vi "SLSC_Engine Get Module Name.vi"(6 "Connect timeout (s)":dbl, 8 "error in (no error)":errorcluster, 10 "compiled.settings":T2={"Name"="", "SLSC Name or IP Address"="", "Slot #"=0, "Configuration Data"={"Properties"={"Boolean Properties"=[], "Double Properties"=[], "I32 Properties"=[], "I64 Properties"=[], "String Properties"=[], "U32 Properties"=[], "U64 Properties"=[]}, "Commands"=[], "Reset Commands"=[], "Apply Values on Deployment"=TRUE, "Apply Reset on Undeployment"=TRUE, "Change Commands"=[]}, "SLSC Get/Read Properties"=[], "SLSC Set/Write Properties"=[], "SLSC Dynamic Commands"=[], "Support Modules"=[]}, 11 "Item Ref in":T1 format="%.0x") -> (0 "error out":errorcluster, 1 "SLSC Module Name":string, 2 "compiled.settings out":T2={"Name"="", "SLSC Name or IP Address"="", "Slot #"=0, "Configuration Data"={"Properties"={"Boolean Properties"=[], "Double Properties"=[], "I32 Properties"=[], "I64 Properties"=[], "String Properties"=[], "U32 Properties"=[], "U64 Properties"=[]}, "Commands"=[], "Reset Commands"=[], "Apply Values on Deployment"=TRUE, "Apply Reset on Undeployment"=TRUE, "Change Commands"=[]}, "SLSC Get/Read Properties"=[], "SLSC Set/Write Properties"=[], "SLSC Dynamic Commands"=[], "Support Modules"=[]}, 3 "Item Ref out":T1 format="%.0x")   [LabVIEW 2017, in "SLSC EDS Engine.lvlib"]
uses:
  SLSC EDS Engine.lvlib
  Shared/Compiled.Settings
  Shared/SLSC Static Settings.ctl
  SLSC CD API/SLSC CD Engine/SLSC Dynamic Channel.ctl
  SLSC CD API/SLSC CD Engine/SLSC Datatype.ctl
  <vilib>/NI Veristand/Custom Device API/Custom Device Item Ref.ctl
  SLSC CD API/SLSC CD Engine/SLSC CD Engine.lvlib
  Shared/SLSC EDS Shared.lvlib
  SLSC CD API/SLSC CD Shared/SLSC CD Shared.lvlib
  <vilib>/NI VeriStand/Custom Device API/Custom Device API.lvlib
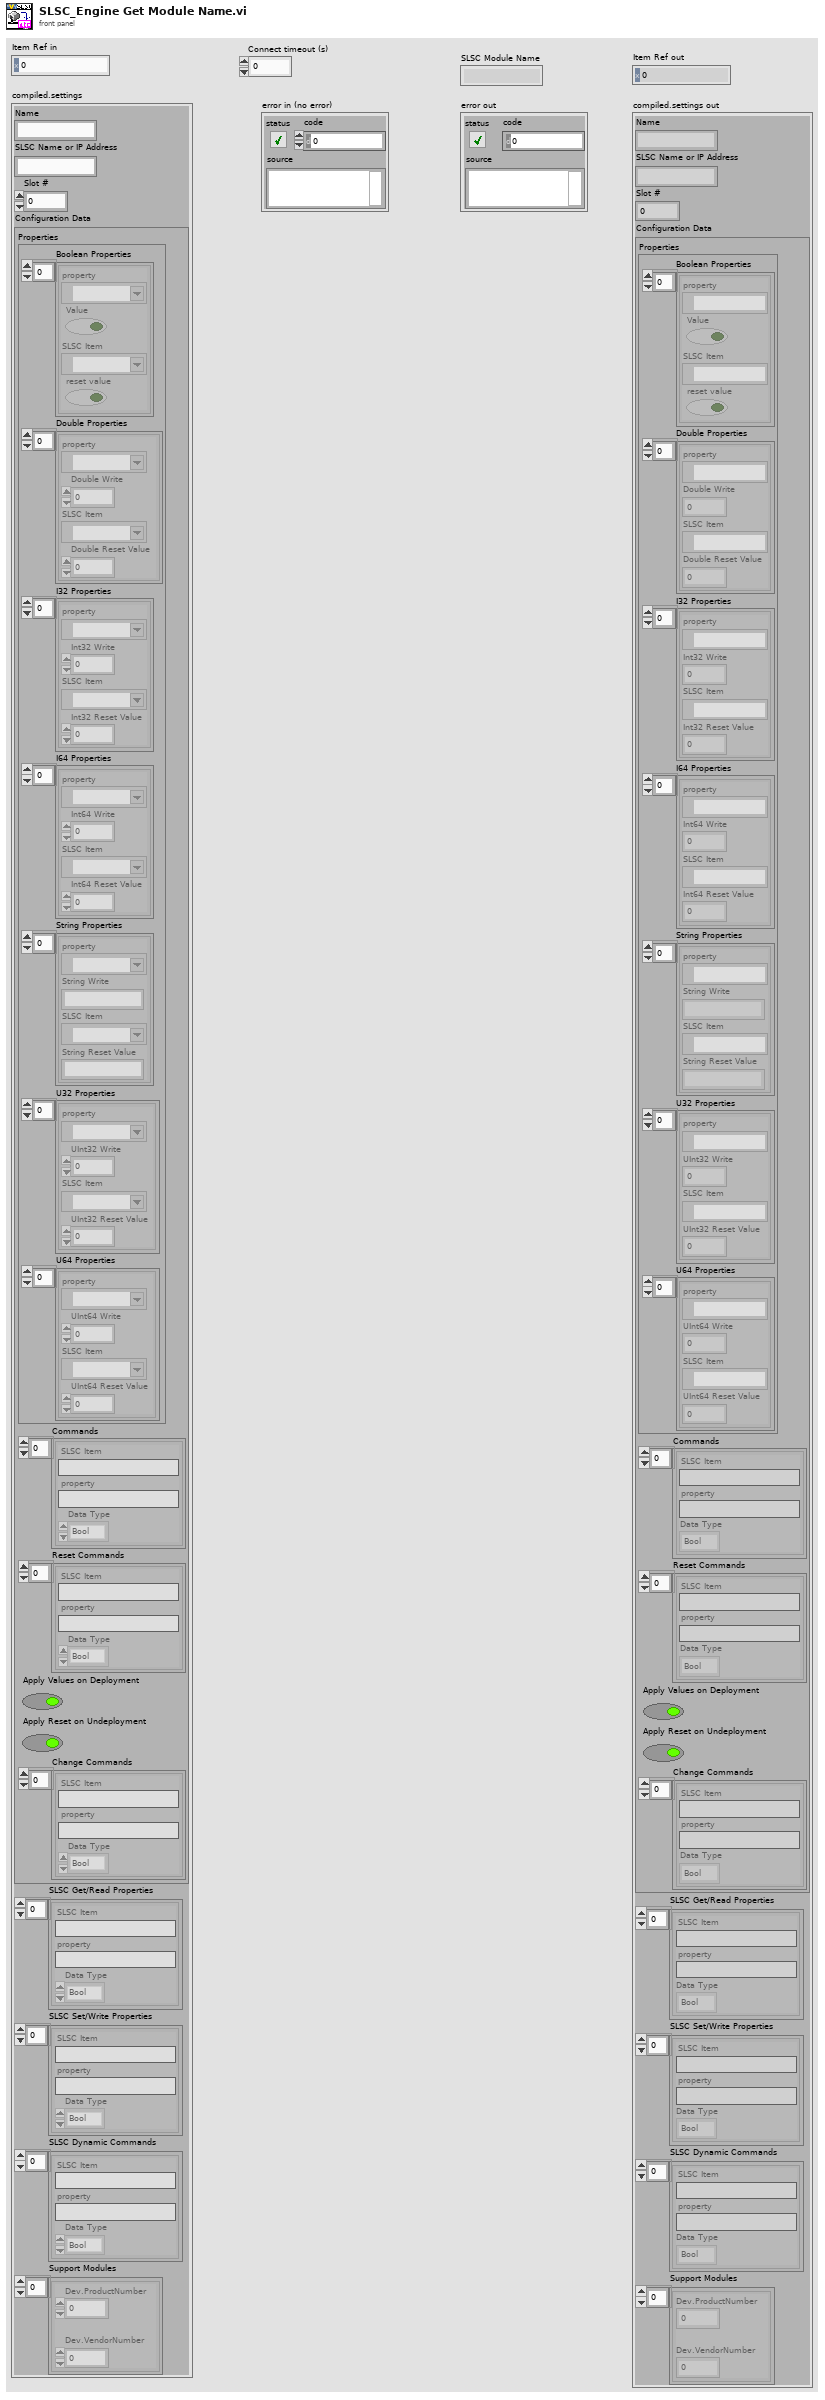
[diagram p1: front panel]
types:
  T1 = typedef "Custom Device API.lvlib/Custom Device Item Ref.ctl" = u64
  T2 = typedef "SLSC EDS Shared.lvlib/Compiled.Settings" = cluster{"Name":string, "SLSC Name or IP Address":string, "Slot #":i32, "Configuration Data":T3, "SLSC Get/Read Properties":T4[], "SLSC Set/Write Properties":T4[], "SLSC Dynamic Commands":T4[], "Support Modules":cluster{"Dev.ProductNumber":u32, "Dev.VendorNumber":u32}[]}
  T3 = typedef "SLSC EDS Shared.lvlib/SLSC Static Settings.ctl" = cluster{"Properties":cluster{"Boolean Properties":cluster{"property":refnum<k21>, "Value":bool, "SLSC Item":refnum<k21>, "reset value":bool}[], "Double Properties":cluster{"property":refnum<k21>, "Double Write":dbl, "SLSC Item":refnum<k21>, "Double Reset Value":dbl}[], "I32 Properties":cluster{"property":refnum<k21>, "Int32 Write":i32, "SLSC Item":refnum<k21>, "Int32 Reset Value":i32}[], "I64 Properties":cluster{"property":refnum<k21>, "Int64 Write":i64, "SLSC Item":refnum<k21>, "Int64 Reset Value":i64}[], "String Properties":cluster{"property":refnum<k21>, "String Write":string, "SLSC Item":refnum<k21>, "String Reset Value":string}[], "U32 Properties":cluster{"property":refnum<k21>, "UInt32 Write":u32, "SLSC Item":refnum<k21>, "UInt32 Reset Value":u32}[], "U64 Properties":cluster{"property":refnum<k21>, "UInt64 Write":u64, "SLSC Item":refnum<k21>, "UInt64 Reset Value":u64}[]}, "Commands":T4[], "Reset Commands":T4[], "Apply Values on Deployment":bool, "Apply Reset on Undeployment":bool, "Change Commands":T4[]}
  T4 = typedef "SLSC CD Shared.lvlib/SLSC Dynamic Channel.ctl" = cluster{"SLSC Item":string, "property":string, "Data Type":T5}
  T5 = typedef "SLSC CD Shared.lvlib/SLSC Datatype.ctl" = enum16{"Bool", "Double", "I32", "I64", "String", "U32", "U64"}
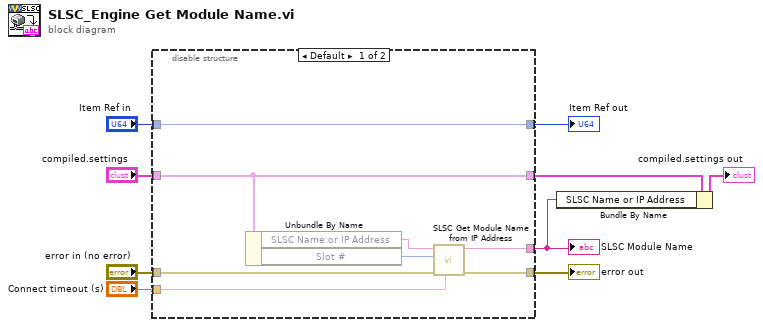
[diagram p0: block diagram]
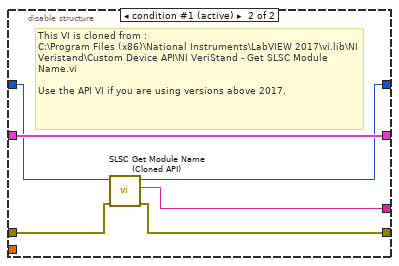
[diagram p2: hidden frame]
diagram:
  n1 = disable-structure shown="Default" {
    disable-tunnel: [w17 w21] -> w2
    disable-tunnel: "error in (no error)" -> [w16 w22]
    disable-tunnel: [w10 w18] -> w1
    disable-tunnel: "compiled.settings" -> [w11 w23]
    disable-tunnel: "Item Ref in" -> [w15 w20]
    disable-tunnel: [w15 w19] -> w6
    disable-tunnel: [w11 w23] -> w9
    disable-tunnel: "Connect timeout (s)" -> [w12 _]
    frame condition #0 {
      n2 = Unbundle By Name(w11) -> ("SLSC Name or IP Address"=w14:string, "Slot #"=w13:i32)
      n3 = call "SLSC Get Module Name from IP Address.vi"("connect timeout"=w12, "Error In"=w16, "Slot #"=w13, "Chassis IP Address"=w14) -> ("Error Out"=w17:errorcluster, "SLSC Module Name"=w10:string)  [unwired: 5 in, 1 out]
    }
    frame condition #1 (active) {
      # "This VI is cloned from :\nC:\\Program Files (x86)\\National Instruments\\LabVIEW 2017\\vi.lib\\NI Veristand\\Custom Device API\\NI VeriStand - Get SLSC Module Name.vi\n\nUse the API VI if you are using versions above 2017."
      n4 = call "SLSC Get Module Name (Cloned API).vi"("error in (no error)"=w22, "Item Ref in"=w20) -> ("error out"=w21:errorcluster, "SLSC Module"=w18:string, "Item Ref out"=w19:T1)  [unwired: 7 in]
    }
  }
  "Item Ref out" <- w6
  "error out" <- w2
  "SLSC Module Name" <- w1
  n5 = Bundle By Name(cluster=w9, "SLSC Name or IP Address"=w1) -> (→"compiled.settings out":T2)
